vi "Fetch VIPM Repo.vi"(8 "error in (no error)":errorcluster, 11 "Repo URL":string="http://download.ni.com/evaluation/labview/lvtn/vipm/") -> (0 "error out":errorcluster, 3 "Repo":refnum<class "Repo.lvclass">)   [LabVIEW 2016, in "Packages.lvlib" / "VIPM.lvlib"]
uses:
  VIPM.lvlib
  Repo_class/Repo.lvclass
  Repo_class/RepoType--enum.ctl
  Repo_class/Repo.lvclass/Repo.ctl
  Package_class/Package.lvclass
  Package Version_class/Package Version.lvclass/Package Version.ctl
  Package_class/Package.lvclass/Package.ctl
  Package Version_class/Read DisplayName.vi
  Package_class/Write Name.vi
  Package_class/Write RepoName.vi
  Package_class/Write RepoType.vi
  Package_class/Write DisplayName.vi
  Package_class/Write Versions.vi
  Repo_class/Write URL.vi
  Repo_class/Write RepoType.vi
  Repo_class/Read Name.vi
  Repo_class/Write Packages.vi
  <vilib>/httpClient/LabVIEWHTTPClient.lvlib
  WSsupport/WSsupport.lvlib
  <vilib>/zip/NI_Unzip.lvlib
  <vilib>/Utility/config.llb/NI_LVConfig.lvlib
  Package Version_class/Package Version.lvclass
panel:
  out "Progress":u8(slide) scale=0.0..100.0
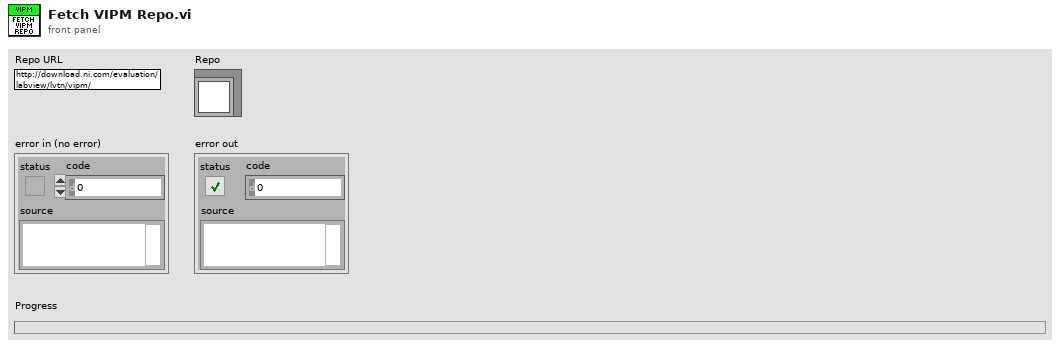
[diagram p1: front panel]
types:
  T1 = typedef "Packages.lvlib/Repo.lvclass/RepoType--enum.ctl" = enum16{"VIPM", "NIPM", "GPM"}
  T2 = typedef "Packages.lvlib/Package--cluster.ctl" = cluster{"Name":string, "Versions":string[]}
  T3 = typedef "NI_LVConfig.lvlib/Config Data RefNum.ctl" = refnum<k1>
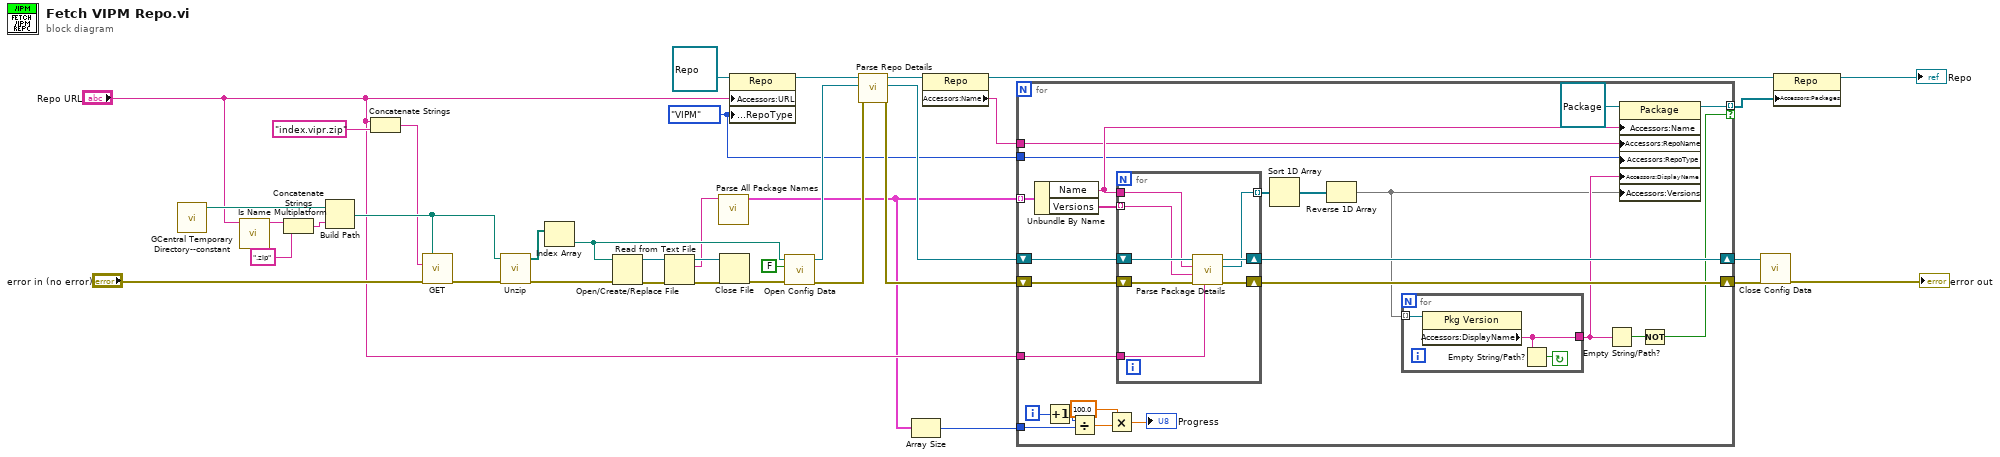
[diagram p0: block diagram]
diagram:
  w3 = RepoType--enum."VIPM" ("RepoType")
  n1 = call "GCentral Temporary Directory--constant.vi"() -> ("GCentral Temporary Directory"=w13:path)  [unwired: 11 in]
  n2 = call <vilib>:"Is Name Multiplatform.vi"("filename"="Repo URL") -> ("suggested filename"=w8:string)  [unwired: 6 in, 4 out]
  n3 = Concatenate Strings(w8, ".zip" ("string")) -> (w7:string)
  n4 = Build Path(base path=w13, name or relative path=w7) -> (appended path=w35:path)
  n5 = Concatenate Strings("Repo URL", "index.vipr.zip" ("string")) -> (w27:string)
  n6 = call <vilib>:"GET.vi"("output file"=w35, "url"=w27, "error in (no error)"="error in (no error)") -> ("error out"=w36:errorcluster)  [unwired: 9 in, 3 out]
  n7 = call <vilib>:"Unzip.vi"("error in (no error)"=w36, "Zip file"=w35) -> ("error out"=w33:errorcluster, "Unzipped files"=w34:path[])  [unwired: 7 in, 1 out]
  n8 = Index Array(array=w34) -> (element=w25:path)  [unwired: 1 in]
  n9 = Open/Create/Replace File(file path (use dialog)=w25, error in=w33) -> (refnum out=w31:refnum<file>, error out=w32:errorcluster)  [unwired: 4 in, 1 out]
  n10 = Read from Text File(file (use dialog)=w31, error in=w32) -> (refnum out=w30:refnum<file>, text=w23:string, error out=w29:errorcluster)  [unwired: 2 in, 1 out]
  n11 = call "Parse All Package Names.vi"("index.vipr"=w23) -> ("All Packages"=w5:T2[])  [unwired: 10 in]
  n12 = Close File(refnum=w30, error in=w29) -> (error out=w26:errorcluster)  [unwired: 1 out]
  n13 = property class="Repo"(reference=refnum<class "Repo.lvclass"> refnum ("Packages.lvlib:Repo"), "Accessors:URL"="Repo URL", "Accessors:RepoType"=w3) -> (reference out=w17:refnum<class "Repo.lvclass">)  [unwired: 1 in, 1 out]
  n14 = call <vilib>:"Open Config Data.vi"("error in (no error)"=w26, "create file if necessary (T)"=FALSE, "configuration file path"=w25) -> ("error out"=w21:errorcluster, "refnum"=w22:T3)  [unwired: 6 in, 1 out]
  n15 = call "Parse Repo Details.vi"("error in (no error)"=w21, "Repo file in"=w22, "Repo in"=w17) -> ("error out"=w18:errorcluster, "Repo file out"=w19:T3, "Repo out"=w12:refnum<class "Repo.lvclass">)  [unwired: 6 in]
  n16 = Array Size(array=w5) -> (size(s)=w4:i32)
  n17 = property class="Repo"(reference=w12) -> (reference out=w2:refnum<class "Repo.lvclass">, "Accessors:Name"=w1:string)  [unwired: 1 in, 1 out]
  n18 = for {
    shift-right: [w59] -> w15
    shift-left: w19 -> [w61]
    shift-right: [w58] -> w14
    shift-left: w18 -> [w60]
    tunnel: w5 -> [w57] mode=indexing
    tunnel: "Repo URL" -> [w55]
    tunnel: [w52] -> w10 mode=indexing if=w40
    tunnel: w4 -> [w50]
    tunnel: w3 -> [w45]
    tunnel: w1 -> [w44]
    i -> [w51]
    n19 = Unbundle By Name(w57) -> ("Name"=w53:string, "Versions"=w56:string[])
    n20 = Increment(x=w51) -> (x+1=w49:i32)
    n21 = Divide(x=w49, y=w50) -> (x/y=w48:dbl)
    n22 = Multiply(x=100.0, y=w48) -> (x*y=→"Progress":dbl)
    n23 = for {
      shift-right: [w69] -> w59
      shift-left: w61 -> [w72]
      shift-right: [w67] -> w58
      shift-left: w60 -> [w71]
      tunnel: w53 -> [w65]
      tunnel: w56 -> [w70] mode=indexing
      tunnel: w55 -> [w68]
      tunnel: [w66] -> w43 mode=indexing
      n24 = call "Parse Package Details.vi"("Repo URL"=w68, "error in (no error)"=w71, "Package Version"=w70, "Package Name"=w65, "Repo file in"=w72) -> ("error out"=w67:errorcluster, "Pkg Version"=w66:refnum<class "Package Version.lvclass">, "Repo file out"=w69:T3)  [unwired: 4 in]
    }
    n25 = Sort 1D Array(array=w43) -> (sorted array=w39:refnum<class "Package Version.lvclass">[])
    n26 = Reverse 1D Array(array=w39) -> (reversed array=w38:refnum<class "Package Version.lvclass">[])
    n27 = for {
      tunnel: [w63] -> w42
      tunnel: w38 -> [w64] mode=indexing
      stop <- w62 continue-if-true
      n28 = property class="Pkg Version"(reference=w64) -> ("Accessors:DisplayName"=w63:string)  [unwired: 1 in, 2 out]
      n29 = Empty String/Path?(string/path=w63) -> (empty?=w62:bool)
    }
    n30 = Empty String/Path?(string/path=w42) -> (empty?=w41:bool)
    n31 = property class="Package"(reference=refnum<class "Package.lvclass"> refnum ("Packages.lvlib:Package"), "Accessors:Name"=w53, "Accessors:RepoName"=w44, "Accessors:RepoType"=w45, "Accessors:DisplayName"=w42, "Accessors:Versions"=w38) -> (reference out=w52:refnum<class "Package.lvclass">)  [unwired: 1 in, 1 out]
    n32 = Not(x=w41) -> (.not. x?=w40:bool)
  }
  n33 = call <vilib>:"Close Config Data.vi"("error in (no error)"=w14, "refnum"=w15) -> ("error out"=→"error out":errorcluster)  [unwired: 8 in, 1 out]
  n34 = property class="Repo"(reference=w2, "Accessors:Packages"=w10) -> (reference out=→"Repo":refnum<class "Repo.lvclass">)  [unwired: 1 in, 1 out]
